vi "Set Direct IO.vi"(8 "error in (no error)":errorcluster, 10 "direct IO":refnum<class "NI_Robotics_Starter Kit Direct IO.lvclass">, 11 "NI_Robotics_Starter Kit Host in":refnum<class "NI_Robotics_Starter Kit Host.lvclass">) -> (0 "error out":errorcluster, 3 "NI_Robotics_Starter Kit Host out":refnum<class "NI_Robotics_Starter Kit Host.lvclass">)   [LabVIEW 2017, in "NI_Robotics_Starter Kit Host.lvclass"]
uses:
  <vilib>/robotics/Starter Kit/Host Interface/NI_Robotics_Starter Kit Host.lvclass
  <vilib>/robotics/Starter Kit/Direct IO/NI_Robotics_Starter Kit Direct IO.lvclass
  <vilib>/robotics/Starter Kit/Host Interface/NI_Robotics_Starter Kit Host.lvclass/NI_Robotics_Starter Kit Host.ctl
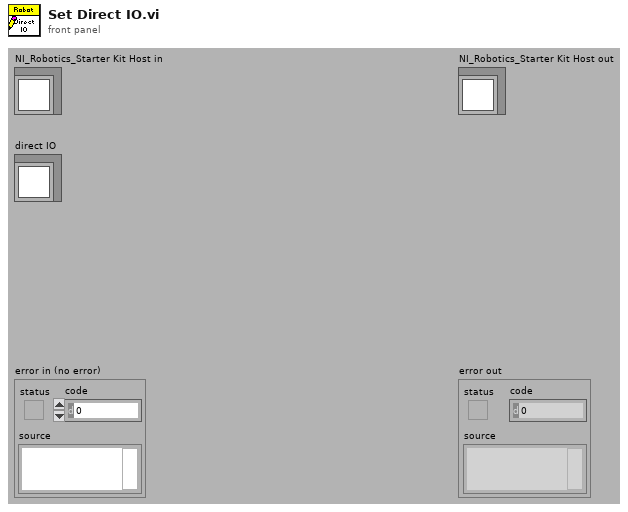
[diagram p1: front panel]
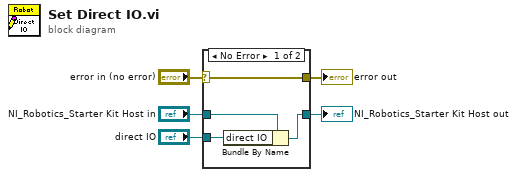
[diagram p0: block diagram]
diagram:
  n1 = case shown="No Error" "error in (no error)" {
    selector: "error in (no error)" -> [w9 w10]
    tunnel: [w9 w10] -> w4
    tunnel: [w7 w11] -> w2
    tunnel: "NI_Robotics_Starter Kit Host in" -> [w8 w11]
    tunnel: "direct IO" -> [w6 _]
    frame No Error {
      n2 = Bundle By Name(cluster=w8, "direct IO"=w6) -> (w7:refnum<class "NI_Robotics_Starter Kit Host.lvclass">)
    }
    frame Error {
    }
  }
  "error out" <- w4
  "NI_Robotics_Starter Kit Host out" <- w2
